vi "Filesaving format_wash.vi"(2 "base path":path=path "C:/Users/TIDAS/OneDrive/AK Tietze/SD", 9 "2D data":dbl[][](array[numeric])=[[-0.35996007919311523, 0.62847900390625, 2.136056900024414, 2.796112060546875, 4.084574222564697, 4.744154453277588, 5.3994526863098145, 6.056264877319336, 7.0342488288879395, 7.692294120788574, 8.35738468170166, 9.340171337127686, 10.849218368530273, 11.509697437286377, 12.170139789581299, 13.766019344329834, 14.743888854980469, 15.400866985321045, 16.061733722686768, 16.721310138702393, 18.25483512878418, 18.918823719024658, 19.57497262954712, 20.235052585601807, 21.52718210220337, 22.183593273162842, 22.839704036712646, 23.4980525970459, 24.473698139190674, 25.129345417022705, 25.7905535697937, 26.77640724182129, 28.283886432647705, 28.94451665878296, 29.602479934692383, 30.26041603088379, 30.917816638946533, 31.575851917266846, 32.2385368347168, 32.89722394943237, 34.41452646255493, 35.075307846069336, 35.73394155502319, 36.39229440689087, 37.68159532546997, 38.33859443664551, 38.99678707122803, 39.65387678146362, 40.629685401916504, 41.286580085754395, 41.94608783721924, 42.60946083068848, 43.26568651199341, 43.92401838302612, 44.58223915100098, 45.8717041015625, 46.848060131073, 47.50630235671997, 48.16454315185547, 48.82181262969971, 50.33476638793945, 0.0, 0.0, 0.0, 0.0, 0.0, 0.0, 0.0, 0.0, 0.0, 0.0, 0.0, 0.0, 0.0, 0.0, 0.0, 0.0, 0.0, 0.0, 0.0, 0.0, 0.0, 0.0, 0.0, 0.0, 0.0, 0.0, 0.0, 0.0, 0.0, 0.0, 0.0, 0.0, 0.0, 0.0, 0.0, 0.0, 0.0, 0.0, 0.0, 0.0, 0.0, 0.0, 0.0, 0.0, 0.0, 0.0, 0.0, 0.0, 0.0, 0.0, 0.0, 0.0, 0.0, 0.0, 0.0, 0.0, 0.0, 0.0, 0.0, 0.0], [0.0, 0.3090169943749474, 0.587785252292473, 0.8090169943749473, 0.9510565162951534, 1.0, 0.9510565162951535, 0.8090169943749476, 0.5877852522924732, 0.30901699437494773, 2.220446049250313e-16, -0.30901699437494706, -0.5877852522924728, -0.8090169943749472, -0.9510565162951534, -1.0, -0.9510565162951536, -0.8090169943749477, -0.5877852522924734, -0.30901699437494795, -3.3306690738754696e-16, 0.30901699437494673, 0.5877852522924728, 0.809016994374947, 0.9510565162951534, 1.0, 0.9510565162951536, 0.8090169943749479, 0.5877852522924734, 0.3090169943749482, 3.3306690738754696e-16, -0.3090169943749466, -0.5877852522924728, -0.8090169943749468, -0.9510565162951534, -0.9999999999999999, -0.9510565162951536, -0.809016994374948, -0.5877852522924734, -0.3090169943749485, -3.3306690738754696e-16, 0.3090169943749462, 0.5877852522924728, 0.8090169943749466, 0.9510565162951534, 0.9999999999999999, 0.9510565162951536, 0.8090169943749482, 0.5877852522924734, 0.3090169943749489, 3.3306690738754696e-16, -0.3090169943749458, -0.5877852522924728, -0.8090169943749463, -0.9510565162951534, -0.9999999999999999, -0.9510565162951536, -0.8090169943749485, -0.5877852522924734, -0.3090169943749493, 0.0, 0.0, 0.0, 0.0, 0.0, 0.0, 0.0, 0.0, 0.0, 0.0, 0.0, 0.0, 0.0, 0.0, 0.0, 0.0, 0.0, 0.0, 0.0, 0.0, 0.0, 0.0, 0.0, 0.0, 0.0, 0.0, 0.0, 0.0, 0.0, 0.0, 0.0, 0.0, 0.0, 0.0, 0.0, 0.0, 0.0, 0.0, 0.0, 0.0, 0.0, 0.0, 0.0, 0.0, 0.0, 0.0, 0.0, 0.0, 0.0, 0.0, 0.0, 0.0, 0.0, 0.0, 0.0, 0.0, 0.0, 0.0, 0.0, 0.0, 0.0], [1311.197, 8055.576000000001, 15491.8, 20690.25, 24095.47, 24838.149999999998, 22980.52, 18617.89, 12391.84, 5233.87, -1559.988, -8405.895, -15263.990000000002, -20208.83, -17455.66, -16578.44, -14762.279999999999, -11138.22, -6530.0019999999995, -2751.14, 3444.0570000000002, 9407.241, 15749.689999999999, 20834.63, 24226.75, 24911.74, 23019.91, 18633.08, 12417.96, 5285.0560000000005, -1511.0349999999999, -8360.875999999998, -15141.84, -19685.95, -20617.829999999998, -18377.6, -15522.8, -11583.199999999999, -6865.657, -3007.1189999999997, 3185.556, 9118.778, 15557.68, 20563.77, 23859.43, 24563.77, 22674.559999999998, 18306.38, 12097.18, 5010.116, -2045.505, -9367.606, -15866.650000000001, -20245.1, -17958.57, -16649.34, -14805.470000000001, -11236.14, -6687.148, -2985.437, 3217.8630000000003, 0.0, 0.0, 0.0, 0.0, 0.0, 0.0, 0.0, 0.0, 0.0, 0.0, 0.0, 0.0, 0.0, 0.0, 0.0, 0.0, 0.0, 0.0, 0.0, 0.0, 0.0, 0.0, 0.0, 0.0, 0.0, 0.0, 0.0, 0.0, 0.0, 0.0, 0.0, 0.0, 0.0, 0.0, 0.0, 0.0, 0.0, 0.0, 0.0, 0.0, 0.0, 0.0, 0.0, 0.0, 0.0, 0.0, 0.0, 0.0, 0.0, 0.0, 0.0, 0.0, 0.0, 0.0, 0.0, 0.0, 0.0, 0.0, 0.0, 0.0]], 10 "Numeric":dbl) -> ()   [LabVIEW 2021]
uses:
  <vilib>/Utility/file.llb/Write Delimited Spreadsheet (DBL).vi
panel:
  in  "0 fM":string="0fM"
  in  "time format string (%c)":string="16112022"
  out "last iteration":dbl
  in  "(indexno.)":i32=1
  out "new file path (Not A Path if cancelled) 2":path=path "C:/Users/TIDAS/OneDrive/AK Tietze/SD/20122021_SD_10^4_UVetched_ATCUN_8_3000fM_HS_1"
  out "resulting string":string="20122021_SD_10^4_UVetched_ATCUN_8_"
  in  "Fluid":string="buffer"
  in  "Membrane No.":string="SE14"
  in  "Peptide":string="ATCUNFAM"
  in  "Membrane Treatment":string="selfetch"
  in  "Pore Denisty":string="10^6"
  in  "Experimentor Initials":string="SD"
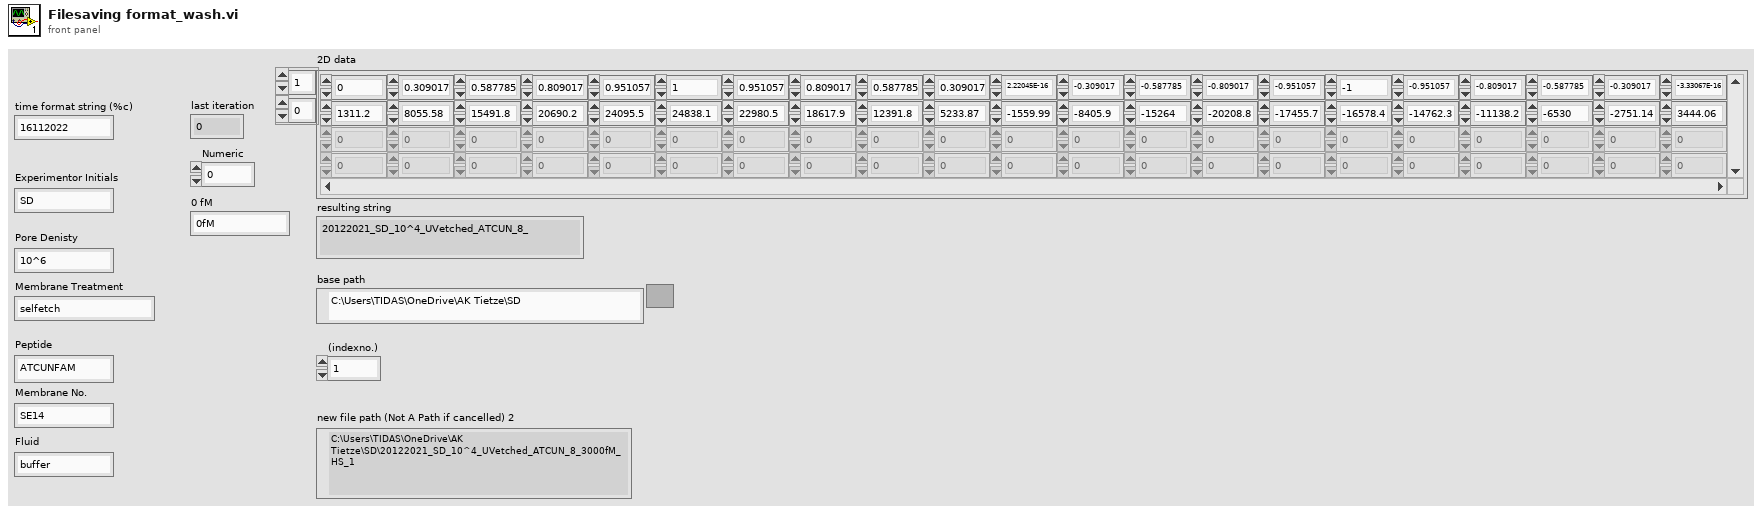
[diagram p1: front panel]
types:
  T1 = enum16{"open", "replace", "create", "open or create", "replace or create", "replace or create with confirmation"}
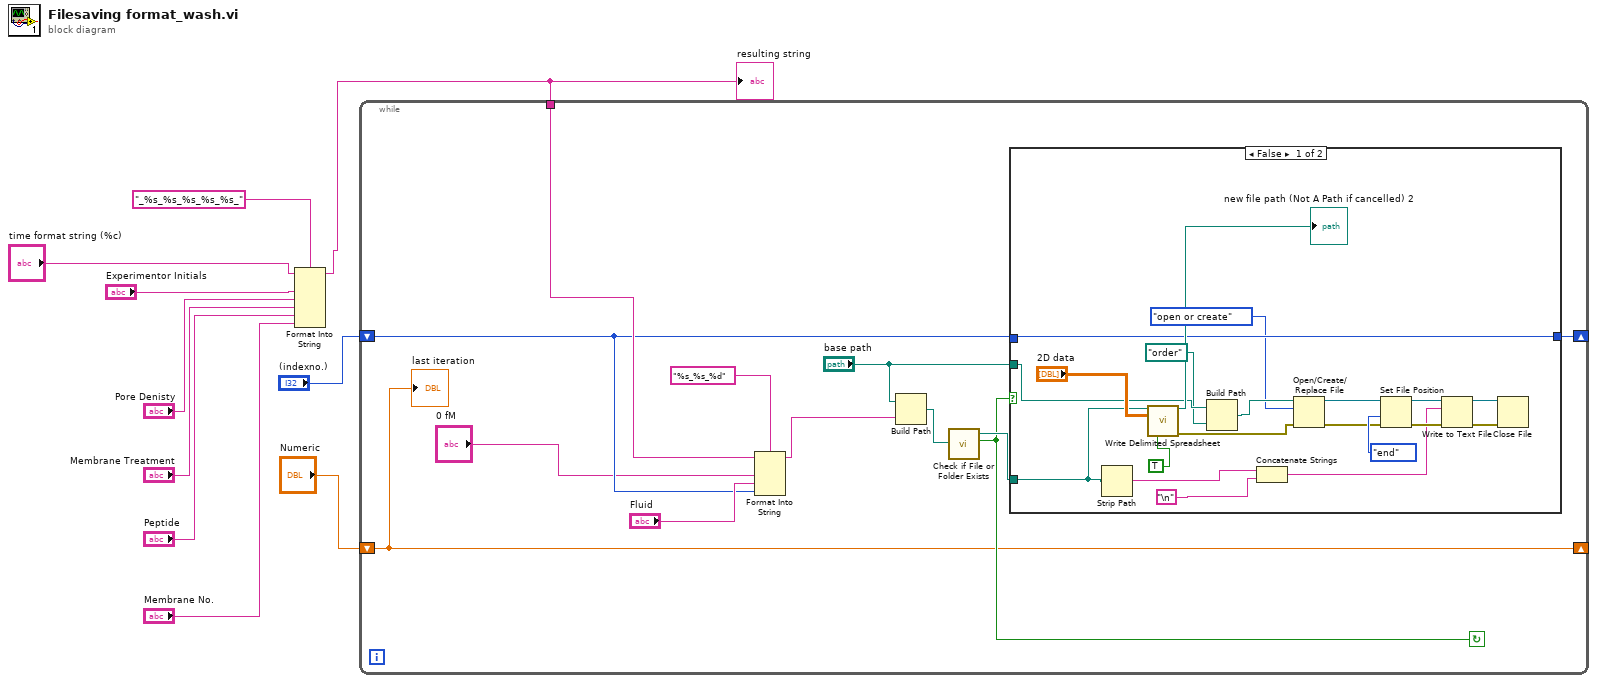
[diagram p0: block diagram]
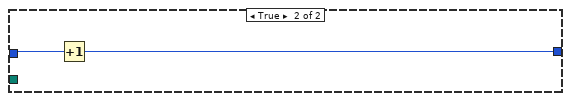
[diagram p2: hidden frame]
diagram:
  n1 = Format Into String(format string="_%s_%s_%s_%s_%s_", initial string="time format string (%c)", "Experimentor Initials", "Pore Denisty", "Membrane Treatment", "Peptide", "Membrane No.") -> (resulting string=w4:string)  [unwired: 1 in, 1 out]
  "resulting string" <- w4
  n2 = while {
    tunnel: w4 -> [w20]
    shift-right: [w13] -> _
    shift-left: "Numeric" -> [w13]
    shift-right: [w14] -> _
    shift-left: "(indexno.)" -> [w15]
    stop <- w16 continue-if-true
    n3 = Format Into String(format string="%s_%s_%d", initial string=w20, "0 fM", "Fluid", w15) -> (resulting string=w21:string)  [unwired: 1 in, 1 out]
    n4 = Build Path(base path="base path", name or relative path=w21) -> (appended path=w18:path)
    n5 = call <vilib>:"Check if File or Folder Exists.vi"("path"=w18) -> ("file or folder exists?"=w16:bool, "dup path"=w17:path)  [unwired: 8 in, 1 out]
    n6 = case shown="False" w16 {
      tunnel: w17 -> [w25 _]
      tunnel: w15 -> [w39 w44]
      tunnel: [w39 w43] -> w14
      tunnel: "base path" -> [w29 _]
      frame False {
        n7 = Strip Path(path=w25) -> (name=w26:string)  [unwired: 1 out]
        n8 = call-poly <vilib>:"Write Delimited Spreadsheet.vi"("file path (dialog if empty)"=w25, "2D data"="2D data", "transpose? (no:F)"=TRUE) -> ("new file path (Not A Path if cancelled)"=→"new file path (Not A Path if cancelled) 2":path, "error out"=w27:errorcluster)  [unwired: 11 in]
        n9 = Build Path(base path=w29, name or relative path=path "order") -> (appended path=w30:path)
        n10 = Concatenate Strings(w26, "\n" ("Line Feed Constant")) -> (w31:string)
        n11 = Open/Create/Replace File(file path (use dialog)=w30, error in=w27, operation (0:open)=T1."open or create") -> (refnum out=w35:refnum<file>, error out=w34:errorcluster)  [unwired: 3 in, 1 out]
        n12 = Set File Position(refnum=w35, from (0:start)=enum16{"start", "end", "current"}."end", error in=w34) -> (refnum out=w33:refnum<file>, error out=w32:errorcluster)  [unwired: 1 in]
        n13 = Write to Text File(file (use dialog)=w33, text=w31, error in=w32) -> (refnum out=w38:refnum<file>, error out=w37:errorcluster)  [unwired: 1 in, 1 out]
        n14 = Close File(refnum=w38, error in=w37) -> ()  [unwired: 2 out]
      }
      frame True {
        n15 = Increment(x=w44) -> (x+1=w43:i32)
      }
    }
    "last iteration" <- w13
  }
